vi "Current VIs Parents Ref.vi"() -> (1 "Calling VI's reference":refnum<vi>)   [LabVIEW 2011]
doc: "Gets a reference to the parent of the VI calling this function. This is useful for creating reusable VIs that opperate on their parent."
panel:
  # "[OpenG VI Tags] ***Do Not Remove***\nCVS Revision = 1.2\nCVS Revision Date = Tue Nov  4 20:27:18 2003\nPackage = oglib_appcontrol-2.7-1\nDepends ="
  # "Current VIs Parents Reference.vi - Gets a reference to the parent of\nthe VI calling this function.\n\nCopyright (C) 2002 James Kring jim@jimkring.com\n\nPlease visit http://www.OpenG.org to learn about the\nOpen Source LabVIEW software movement.\n\nThis library is free software; you can redistribute it and/or\nmodify it under the terms of the GNU Lesser General Public\nLicense as published by the Free Software Foundation; either\nversion 2.1 of the License, or (at your option) any later version.\nThis library is distributed in the hope that it will be useful,\nbut WITHOUT ANY WARRANTY; without even the implied warranty of\nMERCHANTABILITY or FITNESS FOR A PARTICULAR PURPOSE. See the GNU\nLesser General Public License for more details.\nYou should have received a copy of the GNU Lesser General Public\nLicense along with this library; if not, write to the Free Software\nFoundation, Inc., 59 Temple Place, Suite 330, Boston, MA 02111-1307 USA"
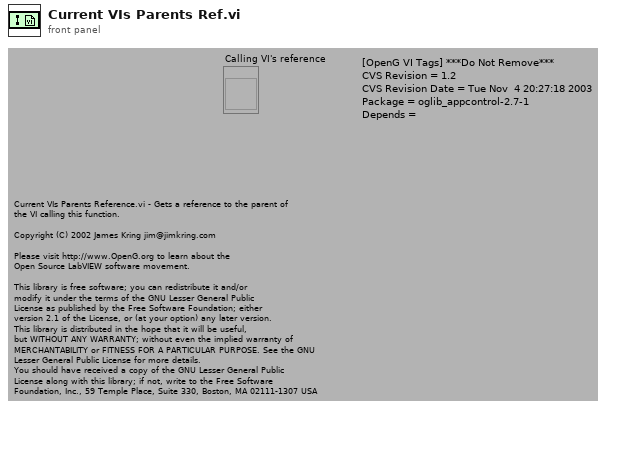
[diagram p1: front panel]
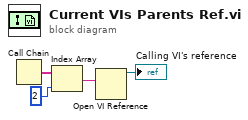
[diagram p0: block diagram]
diagram:
  n1 = Call Chain() -> (call chain=w4:string[])
  n2 = Index Array(array=w4, index=2 ("Index")) -> (element=w2:string)
  n3 = Open VI Reference(vi path=w2) -> (vi reference=→"Calling VI's reference":refnum<vi>)  [unwired: 1 in, 5 out]
